vi "Historian.vi"(4 "Settings":cluster{"Numeric":dbl, "Boolean":bool}, 6 "Initial Time Stamp":timestamp, 7 "Stage":dbl, 8 "error in (no error)":errorcluster, 9 "Sampling Rates":dbl[](array[numeric]), 10 "Sample":dbl, 11 "Path In":path) -> (0 "error out":errorcluster, 2 "Reports":cluster{"Numeric":dbl, "Boolean":bool}, 3 "Path Out":path)   [LabVIEW 2018]
panel:
  in  "Current Time Stamp":timestamp
  in  "Stage Done":bool
  out "Take Sample":bool
  out "Current Stage":dbl
  out "Time of Last Sample":timestamp
  out "Stage Sample Frequency":dbl
  out "Time of Next Sample":timestamp
  out "Timestamp Array":timestamp[](array[timestamp])
  out "Records Array":dbl[](array[numeric])
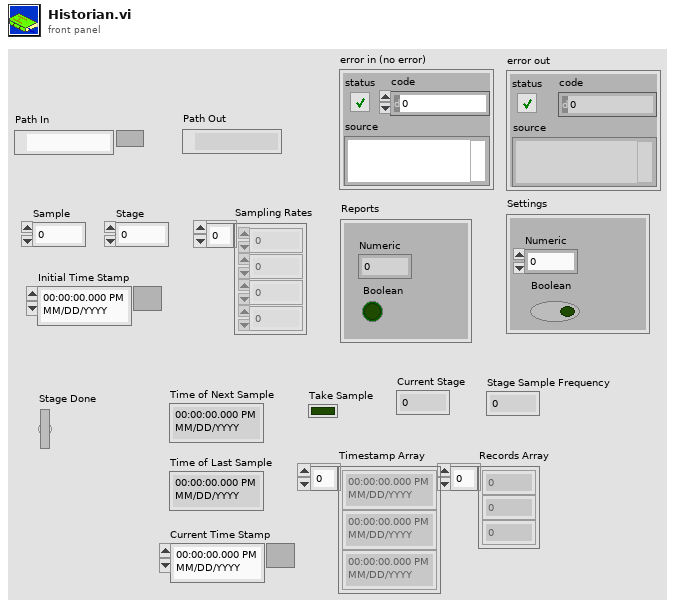
[diagram p1: front panel]
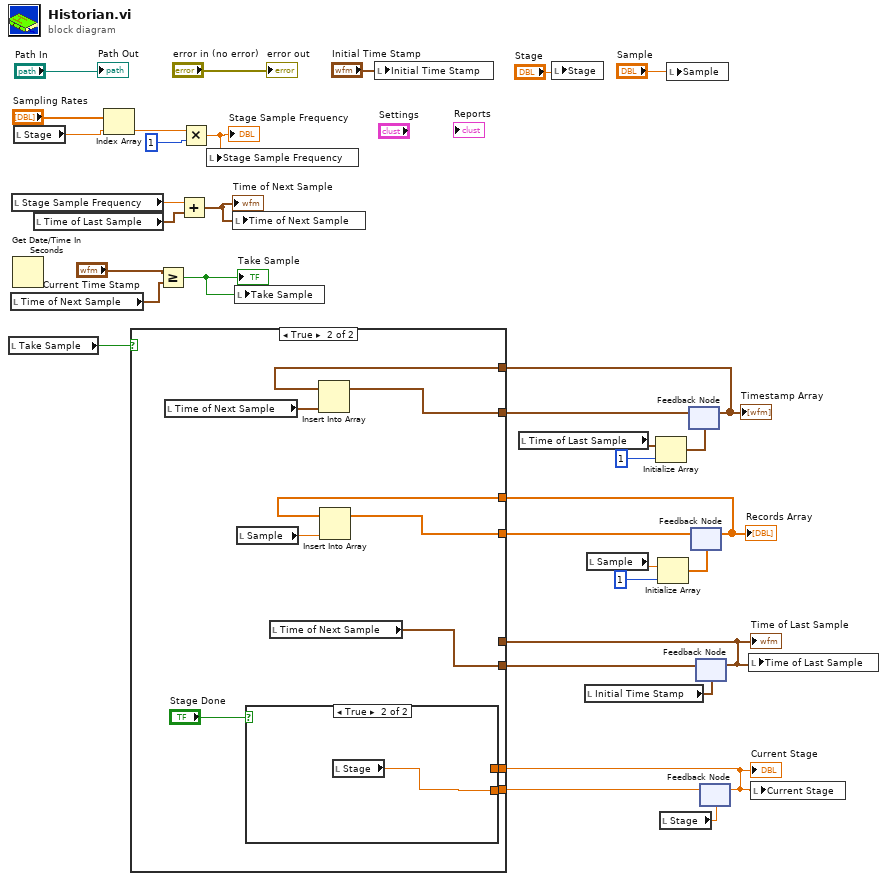
[diagram p0: block diagram]
diagram:
  n1 = local read "Take Sample"() -> (w1:bool)
  n2 = local read "Time of Next Sample"() -> (w21:timestamp)
  n3 = local read "Stage Sample Frequency"() -> (w24:dbl)
  n4 = Get Date/Time In Seconds() -> ()  [unwired: 1 out]
  n5 = local read "Stage"() -> (w20:dbl)
  n6 = local read "Time of Last Sample"() -> (w23:timestamp)
  n7 = Index Array(array="Sampling Rates", index=w20) -> (element=w29:dbl)
  n8 = Greater Or Equal?(x="Current Time Stamp", y=w21) -> (x >= y?=w19:bool)
  "Take Sample" <- w19
  n9 = Add(x=w24, y=w23) -> (x+y=w22:timestamp)
  "Time of Next Sample" <- w22
  n10 = Multiply(x=w29, y=1) -> (x*y=w28:dbl)
  "Stage Sample Frequency" <- w28
  n11 = local write "Stage Sample Frequency"(w28) -> ()
  n12 = local write "Time of Next Sample"(w22) -> ()
  n13 = local write "Take Sample"(w19) -> ()
  n14 = local write "Initial Time Stamp"("Initial Time Stamp") -> ()
  n15 = local read "Time of Last Sample"() -> (w15:timestamp)
  n16 = local write "Stage"("Stage") -> ()
  n17 = local read "Initial Time Stamp"() -> (w13:timestamp)
  n18 = local read "Sample"() -> (w14:dbl)
  n19 = Initialize Array(w15, 1) -> (w26:timestamp[])
  n20 = Initialize Array(w14, 1) -> (w25:dbl[])
  n21 = local read "Stage"() -> (w12:dbl)
  n22 = local write "Sample"("Sample") -> ()
  n23 = feedback #1(w26) -> (w11:timestamp[])
  "Timestamp Array" <- w11
  n24 = feedback #2(w25) -> (w10:dbl[])
  "Records Array" <- w10
  n25 = feedback #3(w13) -> (w9:timestamp)
  "Time of Last Sample" <- w9
  n26 = feedback #4(w12) -> (w8:dbl)
  "Current Stage" <- w8
  n27 = case shown="True" w1 {
    tunnel: w11 -> [w37 w47]
    tunnel: w10 -> [w36 w46]
    tunnel: w9 -> [w35 _]
    tunnel: w8 -> [w34 w42]
    tunnel: [w37 w45] -> w7
    tunnel: [w36 w44] -> w6
    tunnel: [w35 w40] -> w5
    tunnel: [w34 w41] -> w4
    frame False {
    }
    frame True {
      n28 = local read "Time of Next Sample"() -> (w39:timestamp)
      n29 = local read "Sample"() -> (w38:dbl)
      n30 = case shown="True" "Stage Done" {
        tunnel: w42 -> [w48 _]
        tunnel: [w48 w49] -> w41
        frame False {
        }
        frame True {
          n31 = local read "Stage"() -> (w49:dbl)
        }
      }
      n32 = local read "Time of Next Sample"() -> (w40:timestamp)
      n33 = Insert Into Array(array=w47, new element=w39) -> (w45:timestamp[])  [unwired: 1 in]
      n34 = Insert Into Array(array=w46, new element=w38) -> (w44:dbl[])  [unwired: 1 in]
    }
  }
  n35 = feedback-in #1(w7) -> ()
  n36 = feedback-in #2(w6) -> ()
  n37 = feedback-in #3(w5) -> ()
  n38 = feedback-in #4(w4) -> ()
  n39 = local write "Time of Last Sample"(w9) -> ()
  n40 = local write "Current Stage"(w8) -> ()
  "error out" <- "error in (no error)"
  "Path Out" <- "Path In"
